vi "USB6343_Control_v1.2.5.vi"(9 "event rsg handle":refnum<event-registration>) -> ()   [LabVIEW 2013]
uses:
  <vilib>/DAQmx/read.llb/DAQmx Read.vi
  <vilib>/DAQmx/read.llb/DAQmx Read (Counter DBL 1Chan 1Samp).vi
  <vilib>/DAQmx/write.llb/DAQmx Write.vi
  <vilib>/DAQmx/write.llb/DAQmx Write (Digital 1D Bool NChan 1Samp 1Line).vi
  <vilib>/DAQmx/write.llb/DAQmx Write (Analog 1D DBL NChan 1Samp).vi
  <vilib>/DAQmx/read.llb/DAQmx Read (Analog 1D DBL NChan 1Samp).vi
  <vilib>/DAQmx/miscellaneous.llb/DAQmx Fill In Error Info.vi
panel:
  in  "monitor interface":T1
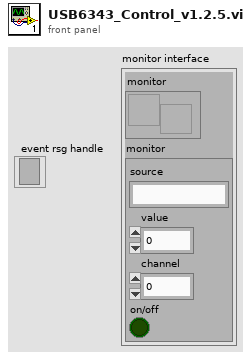
[diagram p1: front panel]
types:
  T1 = cluster{"monitor":refnum<user-event>, "monitor":cluster{"source":string, "value":dbl, "channel":i32, "on/off":bool}}
  T2 = cluster{"AI Task":refnum<k21>, "AO Task":refnum<k21>, "DO Task":refnum<k21>, "DI Task":refnum<k21>}
  T3 = cluster{"source":string, "value":dbl, "channel":i32, "on/off":bool}
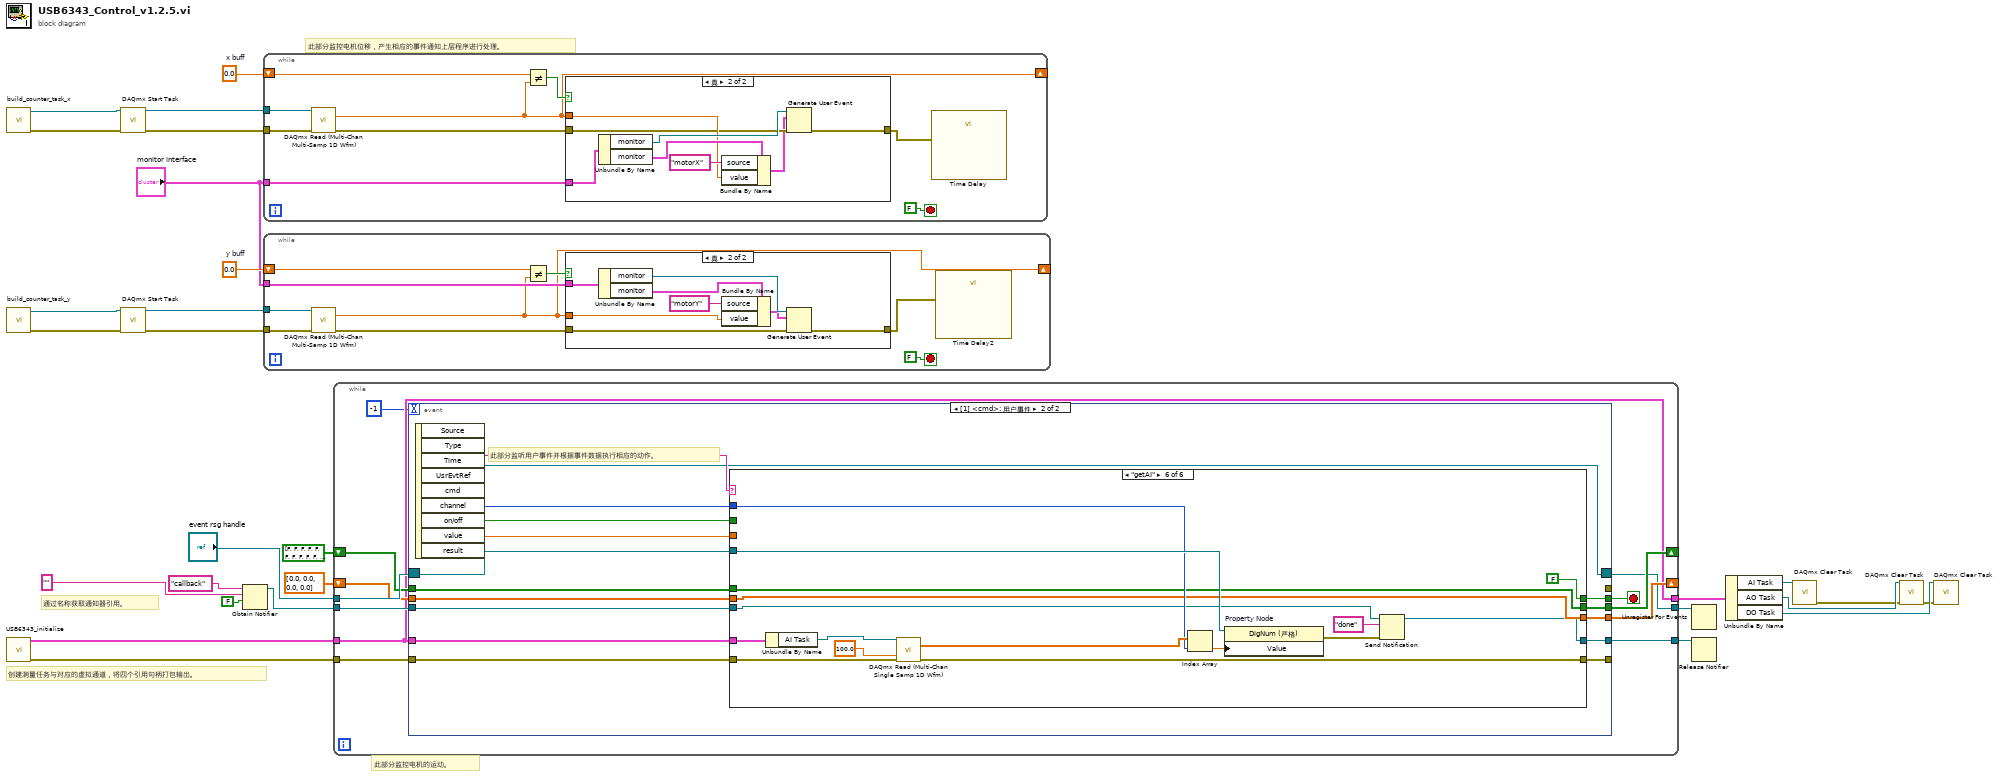
[diagram p0: block diagram]
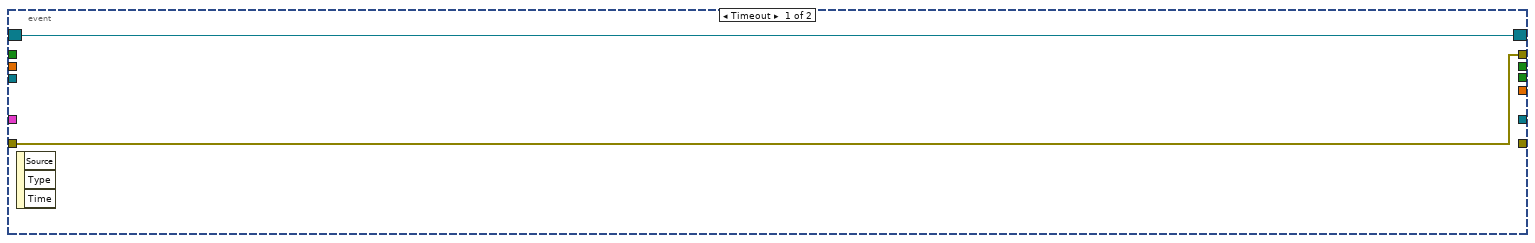
[diagram p4: hidden frame]
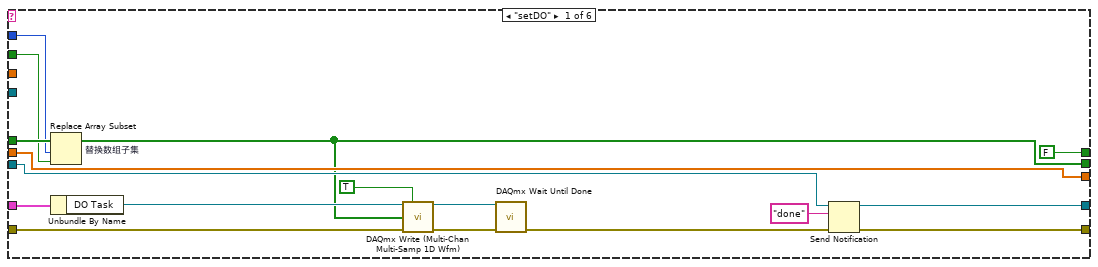
[diagram p5: hidden frame]
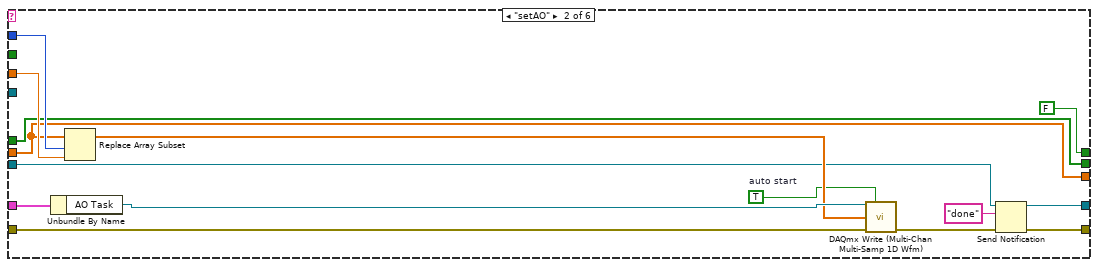
[diagram p6: hidden frame]
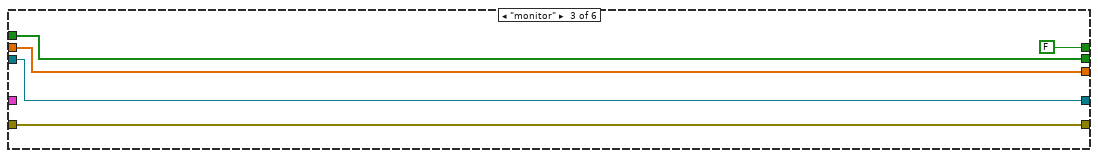
[diagram p7: hidden frame]
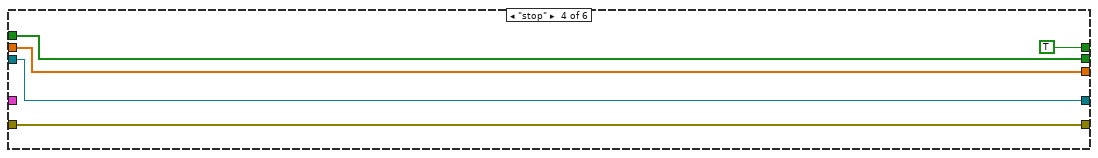
[diagram p8: hidden frame]
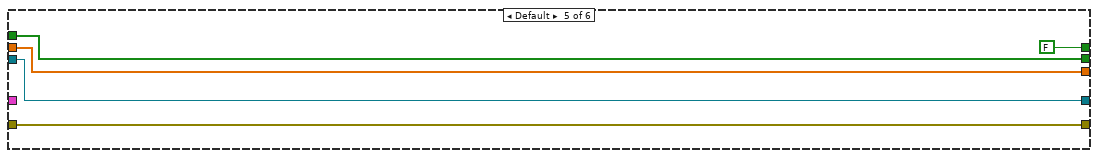
[diagram p9: hidden frame]
diagram:
  w6 = 0.0  # x buff
  w9 = 0.0  # y buff
  # "此部分监控电机位移，产生相应的事件通知上层程序进行处理。"
  # "此部分监控电机的运动。"
  # "通过名称获取通知器引用。"
  # "创建测量任务与对应的虚拟通道，将四个引用句柄打包输出。"
  n1 = call "build_counter_task_x.vi"() -> ("error out"=w5:errorcluster, "task out"=w4:refnum<k21>)  [unwired: 10 in]
  n2 = call "build_counter_task_y.vi"() -> ("error out"=w1:errorcluster, "task out"=w2:refnum<k21>)  [unwired: 10 in]
  n3 = call "USB6343_initialize.vi"() -> ("error out"=w28:errorcluster, "tasks"=w12:T2)  [unwired: 10 in]
  n4 = call <vilib>:"DAQmx Start Task.vi"("task/channels in"=w4, "error in"=w5) -> ("task out"=w8:refnum<k21>, "error out"=w7:errorcluster)  [unwired: 12 in]
  n5 = call <vilib>:"DAQmx Start Task.vi"("task/channels in"=w2, "error in"=w1) -> ("task out"=w11:refnum<k21>, "error out"=w10:errorcluster)  [unwired: 12 in]
  n6 = Obtain Notifier(name (unnamed)="callback" ("名称（未命名）"), notification data type="", create if not found? (T)=FALSE ("如未找到是否创建？(T)")) -> (notifier out=w19:refnum<notifier>)  [unwired: 1 in, 2 out]
  n7 = while {
    tunnel: w8 -> [w34]
    tunnel: w7 -> [w37]
    shift-right: [w32] -> _
    shift-left: w6 -> [w36]
    tunnel: "monitor interface" -> [w35]
    stop <- FALSE stop-if-true
    n8 = call-poly "DAQmx Read (Multi-Chan Multi-Samp 1D Wfm).vi"("task/channels in"=w34, "error in"=w37) -> ("data"=w32:dbl, "error out"=w31:errorcluster)  [unwired: 11 in, 1 out]
    n9 = Not Equal?(x=w36, y=w32) -> (x != y?=w33:bool)
    n10 = case shown="真" w33 {
      tunnel: w35 -> [_ w46]
      tunnel: w32 -> [_ w42]
      tunnel: w31 -> [w38 w41]
      tunnel: [w38 w39] -> w29
      frame False {
      }
      frame True {
        n11 = Unbundle By Name(w46) -> ("monitor"=w45:refnum<user-event>, "monitor"=w44:T3)
        n12 = Bundle By Name(cluster=w44, "source"="motorX", "value"=w42) -> (w40:T3)
        n13 = Generate User Event(user event=w45, event data cluster=w40, error in=w41) -> (error out=w39:errorcluster)  [unwired: 1 in, 1 out]
      }
    }
    n14 = call "Time Delay"("error in (no error)"=w29) -> ()  [unwired: 10 in, 1 out]
  }
  n15 = while {
    tunnel: w11 -> [w52]
    tunnel: w10 -> [w55]
    shift-right: [w50] -> _
    shift-left: w9 -> [w54]
    tunnel: "monitor interface" -> [w53]
    stop <- FALSE stop-if-true
    n16 = call-poly "DAQmx Read (Multi-Chan Multi-Samp 1D Wfm).vi"("task/channels in"=w52, "error in"=w55) -> ("data"=w50:dbl, "error out"=w49:errorcluster)  [unwired: 11 in, 1 out]
    n17 = Not Equal?(x=w54, y=w50) -> (x != y?=w51:bool)
    n18 = case shown="真" w51 {
      tunnel: w53 -> [_ w64]
      tunnel: w50 -> [_ w60]
      tunnel: w49 -> [w56 w59]
      tunnel: [w56 w57] -> w47
      frame False {
      }
      frame True {
        n19 = Unbundle By Name(w64) -> ("monitor"=w63:refnum<user-event>, "monitor"=w62:T3)
        n20 = Bundle By Name(cluster=w62, "source"="motorY", "value"=w60) -> (w58:T3)
        n21 = Generate User Event(user event=w63, event data cluster=w58, error in=w59) -> (error out=w57:errorcluster)  [unwired: 1 in, 1 out]
      }
    }
    n22 = call "Time Delay2"("error in (no error)"=w47) -> ()  [unwired: 10 in, 1 out]
  }
  n23 = while {
    tunnel: w12 -> [w66]
    tunnel: w28 -> [w76]
    tunnel: "event rsg handle" -> [w75]
    shift-right: [w73] -> _
    shift-left: bool[] [FALSE, FALSE, FALSE, FALSE, FALSE, FALSE, FALSE, FALSE, FALSE, FALSE, FALSE, FALSE, FALSE, FALSE, FALSE, FALSE] -> [w74]
    shift-right: [w70] -> _
    shift-left: dbl[] [0.0, 0.0, 0.0, 0.0] ("data") -> [w71]
    tunnel: [w69] -> w23
    tunnel: w19 -> [w68]
    tunnel: [w67] -> w18
    tunnel: [w66] -> w16
    stop <- w72 stop-if-true
    n24 = event shown="[1] <cmd>: 用户事件" {
      selector: w75 -> [w77 w81]
      dyn-events: [w77 w81] -> w69
      timeout: -1 -> [_ _]
      tunnel: w66 -> [_ w93]
      tunnel: [w78 _] -> _
      tunnel: w76 -> [w78 w92]
      tunnel: w74 -> [_ w91]
      tunnel: [_ w89] -> w73
      tunnel: [_ w87] -> w72
      tunnel: w71 -> [_ w86]
      tunnel: [_ w84] -> w70
      tunnel: [_ w82] -> _
      tunnel: w68 -> [_ w80]
      tunnel: [_ w79] -> w67
      event Timeout {
        n25 = event-data() -> ()  [unwired: 1 in, 3 out]
      }
      event User Event {
        # "此部分监听用户事件并根据事件数据执行相应的动作。"
        n26 = event-data() -> ("cmd"=w88:string, "channel"=w94:i32, "on/off"=w90:bool, "value"=w85:dbl, "result"=w83:refnum<vi>)  [unwired: 1 in, 4 out]
        n27 = case shown="\"getAI\"" w88 {
          tunnel: w94 -> [w109 w124 _ _ _ w151]
          tunnel: w93 -> [w111 w126 _ _ _ w157]
          tunnel: w92 -> [w101 w117 w128 w133 w138 w153]
          tunnel: w91 -> [w110 w121 w131 w136 w141 w149]
          tunnel: w90 -> [w108 _ _ _ _ _]
          tunnel: [w99 w121 w131 w136 w141 w149] -> w89
          tunnel: [FALSE FALSE FALSE TRUE FALSE FALSE] -> w87
          tunnel: w86 -> [w106 w122 w130 w134 w139 w148]
          tunnel: w85 -> [_ w123 _ _ _ _]
          tunnel: [w106 w122 w130 w134 w139 w148] -> w84
          tunnel: w83 -> [_ _ _ _ _ w155]
          tunnel: [w105 w115 w128 w133 w138 w146] -> w82
          tunnel: w80 -> [w104 w113 w127 w132 w137 w145]
          tunnel: [w102 w114 w127 w132 w137 w144] -> w79
          frame "setDO" {
            n28 = Replace Array Subset "替换数组子集"(array=w110, new element=w108, index=w109) -> (w99:bool[])
            n29 = Unbundle By Name(w111) -> ("DO Task"=w100:refnum<k21>)
            n30 = call-poly "DAQmx Write (Multi-Chan Multi-Samp 1D Wfm).vi"("task/channels in"=w100, "auto start"=TRUE, "data"=w99, "error in"=w101) -> ("task out"=w95:refnum<k21>, "error out"=w97:errorcluster)  [unwired: 9 in, 1 out]
            n31 = call <vilib>:"DAQmx Wait Until Done.vi"("task/channels in"=w95, "error in"=w97) -> ("error out"=w96:errorcluster)  [unwired: 12 in, 1 out]
            n32 = Send Notification(notification="done" ("通知"), notifier=w104, error in (no error)=w96) -> (notifier out=w102:refnum<notifier>, error out=w105:errorcluster)
          }
          frame "setAO" {
            w119 = TRUE  # auto start
            n33 = Unbundle By Name(w126) -> ("AO Task"=w125:refnum<k21>)
            n34 = Replace Array Subset(array=w122, new element=w123, index=w124) -> (w120:dbl[])
            n35 = call-poly "DAQmx Write (Multi-Chan Multi-Samp 1D Wfm).vi"("task/channels in"=w125, "auto start"=w119, "data"=w120, "error in"=w117) -> ("error out"=w116:errorcluster)  [unwired: 9 in, 2 out]
            n36 = Send Notification(notification="done" ("通知"), notifier=w113, error in (no error)=w116) -> (notifier out=w114:refnum<notifier>, error out=w115:errorcluster)
          }
          frame "monitor" {
          }
          frame "stop" {
          }
          frame Default {
          }
          frame "getAI" {
            n37 = Unbundle By Name(w157) -> ("AI Task"=w156:refnum<k21>)
            n38 = call-poly "DAQmx Read (Multi-Chan Single Samp 1D Wfm).vi"("task/channels in"=w156, "timeout"=100.0, "error in"=w153) -> ("data"=w152:dbl[], "error out"=w146:errorcluster)  [unwired: 10 in, 1 out]
            n39 = Index Array(array=w152, index=w151) -> (element=w150:dbl)
            n40 = property on="Property Node" class="DigNum (严格)"(reference=w155, "Value"=w150) -> (error out=w142:errorcluster)  [unwired: 1 in, 1 out]
            n41 = Send Notification(notification="done" ("通知"), notifier=w145, error in (no error)=w142) -> (notifier out=w144:refnum<notifier>)  [unwired: 1 out]
          }
        }
      }
    }
  }
  n42 = Unregister For Events(event registration refnum=w23) -> ()  [unwired: 1 in, 1 out]
  n43 = Release Notifier(notifier=w18) -> ()  [unwired: 2 in, 3 out]
  n44 = Unbundle By Name(w16) -> ("AI Task"=w27:refnum<k21>, "AO Task"=w26:refnum<k21>, "DO Task"=w25:refnum<k21>)
  n45 = call <vilib>:"DAQmx Clear Task.vi"("task in"=w27) -> ("error out"=w15:errorcluster)  [unwired: 14 in]
  n46 = call <vilib>:"DAQmx Clear Task.vi"("task in"=w26, "error in"=w15) -> ("error out"=w14:errorcluster)  [unwired: 13 in]
  n47 = call <vilib>:"DAQmx Clear Task.vi"("task in"=w25, "error in"=w14) -> ()  [unwired: 13 in, 1 out]
